vi "STARTUP_.vi"() -> ()   [LabVIEW 2015]
panel:
  out "Current Startup\nAttempt Case - Right 2":i32
  in  "LEFT FOUND":bool
  in  "RIGHT FOUND":bool
  in  "Left Start\nCorrelation Score":dbl
  in  "Right Start\nCorrelation Score":dbl
  out "Current Startup\nAttempt Case - Right":i32
  out "Current Startup\nAttempt Case - Left":i32
  out "Start up Template State\n- LEFT":i32
  in  "Skip Startup - LEFT":bool[](array[boolean])=[FALSE, TRUE, FALSE, FALSE, TRUE, FALSE, FALSE, TRUE]
  in  "Skip Startup - RIGHT":bool[](array[boolean])=[TRUE, TRUE, FALSE, FALSE, FALSE, FALSE, FALSE, FALSE]
  in  "Startup GP per Case - LEFT":u16[](array[numeric])=[920, 0, 260, 700, 0, 200, 650, 0, 358]
  in  "Startup GP per Case - RIGHT":u16[](array[numeric])=[0, 0, 360, 830, 130, 340, 790, 0]
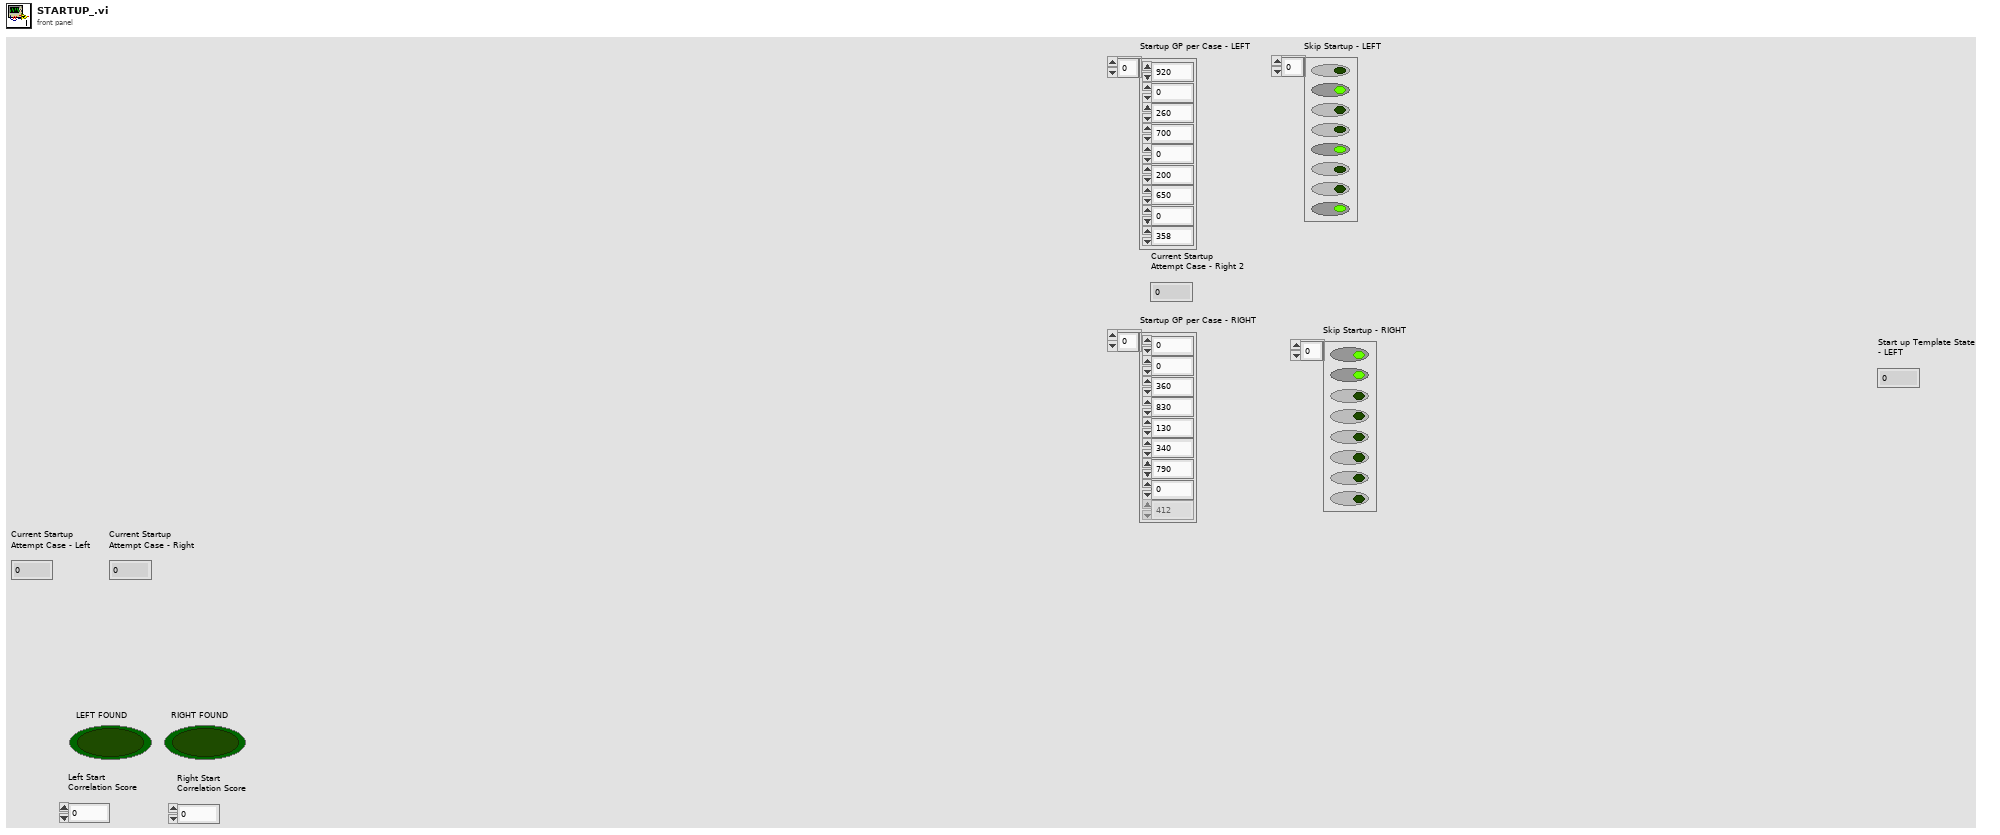
[diagram p1: front panel]
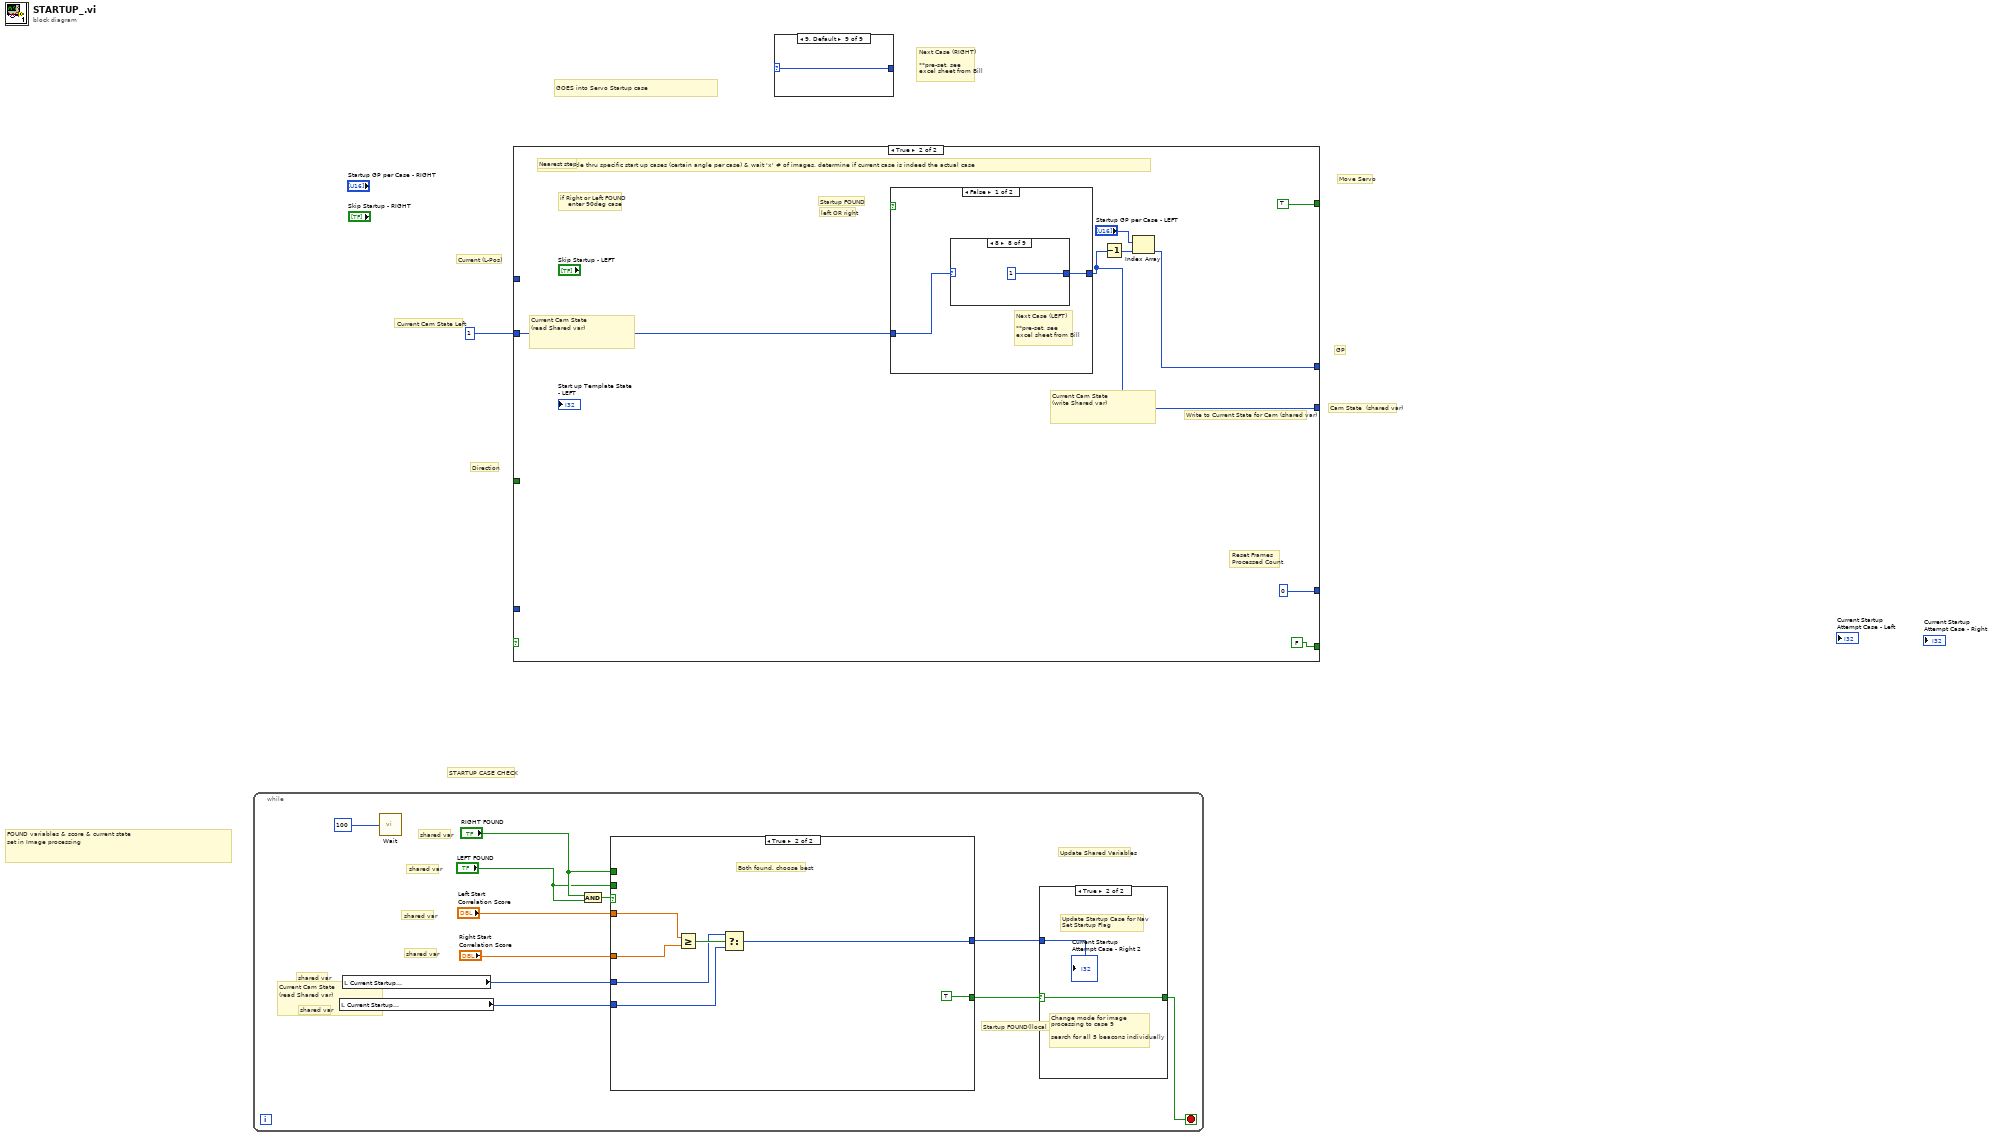
[diagram p0: block diagram]
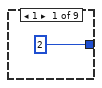
[diagram p2: hidden frame]
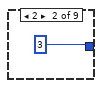
[diagram p3: hidden frame]
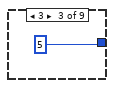
[diagram p4: hidden frame]
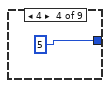
[diagram p5: hidden frame]
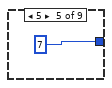
[diagram p6: hidden frame]
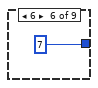
[diagram p7: hidden frame]
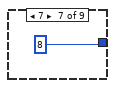
[diagram p8: hidden frame]
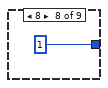
[diagram p9: hidden frame]
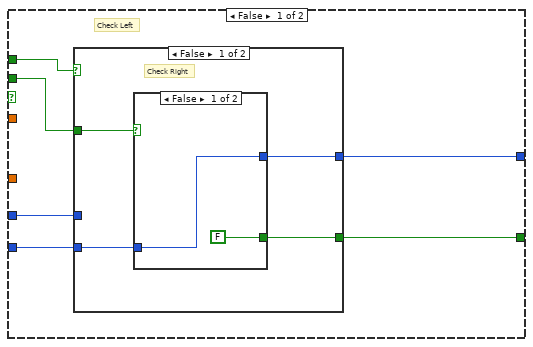
[diagram p11: hidden frame]
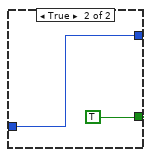
[diagram p12: hidden frame]
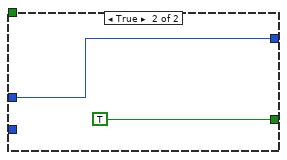
[diagram p13: hidden frame]
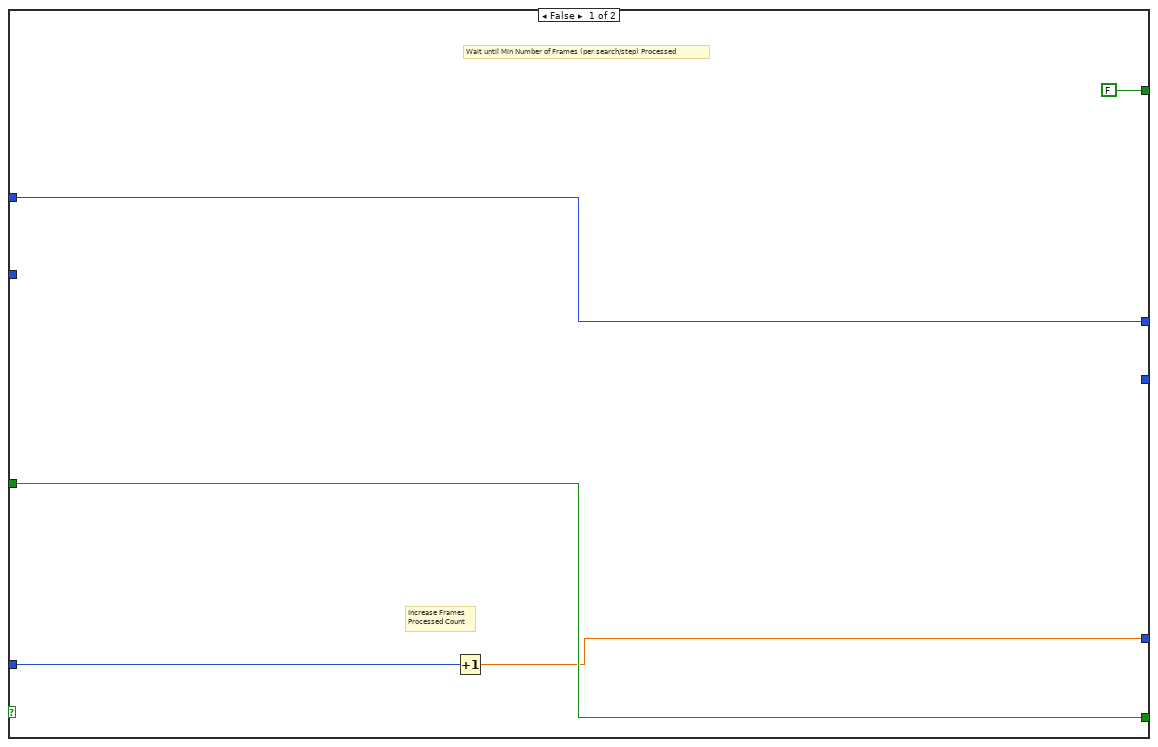
[diagram p14: hidden frame]
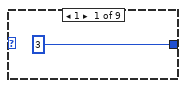
[diagram p15: hidden frame]
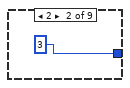
[diagram p16: hidden frame]
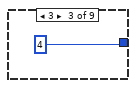
[diagram p17: hidden frame]
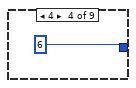
[diagram p18: hidden frame]
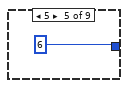
[diagram p19: hidden frame]
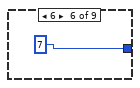
[diagram p20: hidden frame]
diagram:
  # "Next Case (RIGHT)\n\n**pre-set, see\nexcel sheet from Bill"
  # "Cam State  (shared var)"
  # "FOUND variables & score & current state\nset in Image processing"
  # "GOES into Servo Startup case"
  # "STARTUP CASE CHECK"
  # "GP"
  # "Move Servo"
  # "Current Cam State Left"
  # "Direction"
  # "Current (L-Pos)"
  n1 = while {
    stop <- w2 stop-if-true
    # "Startup FOUND(llocal var)"
    # "Current Cam State\n(read Shared var)"
    # "shared var"
    # "shared var"
    # "shared var"
    # "shared var"
    # "shared var"
    # "shared var"
    # "Update Shared Variables"
    n2 = local read "Current Startup\nAttempt Case - Right"() -> (w9:i32)
    n3 = local read "Current Startup\nAttempt Case - Left"() -> (w10:i32)
    n4 = call "Wait"("Count(mSec)"=u32 100) -> ()  [unwired: 1 out]
    n5 = And(x="RIGHT FOUND", y="LEFT FOUND") -> (x .and. y?=w8:bool)
    n6 = case shown="True" w8 {
      tunnel: "Left Start\nCorrelation Score" -> [_ w36]
      tunnel: "Right Start\nCorrelation Score" -> [_ w38]
      tunnel: w10 -> [w19 w35]
      tunnel: w9 -> [w17 w34]
      tunnel: [w20 w33] -> w4
      tunnel: "RIGHT FOUND" -> [w21 _]
      tunnel: "LEFT FOUND" -> [w18 _]
      tunnel: [w16 TRUE] -> w5
      frame False {
        # "Check Left"
        n7 = case shown="False" w21 {
          tunnel: [w24 w31] -> w20
          tunnel: w19 -> [_ w31]
          tunnel: w18 -> [w25 _]
          tunnel: w17 -> [w23 _]
          tunnel: [w22 TRUE] -> w16
          frame False {
            # "Check Right"
            n8 = case shown="False" w25 {
              tunnel: [w26 w29] -> w24
              tunnel: w23 -> [w26 w29]
              tunnel: [FALSE TRUE] -> w22
              frame False {
              }
              frame True {
              }
            }
          }
          frame True {
          }
        }
      }
      frame True {
        # "Both found, choose best"
        n9 = Greater Or Equal?(x=w36, y=w38) -> (x >= y?=w37:bool)
        n10 = Select(t=w35, s=w37, f=w34) -> (s? t:f=w33:i32)
      }
    }
    n11 = case shown="True" w5 {
      selector: w5 -> [w13 w15]
      tunnel: w4 -> [_ w14]
      tunnel: [w13 w15] -> w2
      frame False {
        # "Do nothing"
      }
      frame True {
        # "Change mode for image\nprocessing to case 9\n\nsearch for all 5 beacons individually"
        # "Update Startup Case for Nav\nSet Startup Flag"
        "Current Startup\nAttempt Case - Right 2" <- w14
      }
    }
  }
  n12 = case shown="True" {
    selector: _ -> [_ _]
    tunnel: _ -> [w41 _]
    tunnel: _ -> [w40 _]
    tunnel: [w41 w45] -> _
    tunnel: [w39 0] -> _
    tunnel: [FALSE TRUE] -> _
    tunnel: _ -> [w42 _]
    tunnel: [w40 FALSE] -> _
    tunnel: 1 -> [_ w48]
    tunnel: [_ w44] -> _
    frame False {
      # "Wait until Min Number of Frames (per search/step) Processed"
      # "Increase Frames\nProcessed Count"
      n13 = Increment(x=w42) -> (x+1=w39:dbl)
    }
    frame True {
      # "left OR right"
      # "Startup FOUND"
      # "Current Cam State\n(write Shared var)"
      # "Current Cam State\n(read Shared var)"
      # "Write to Current State for Cam (shared var)"
      # "if Right or Left FOUND\n    enter 90deg case"
      # "Reset Frames\nProcessed Count"
      # "Startup - Cycle thru specific start up cases (certain angle per case) & wait 'x' # of images, determine if current case is indeed the actual case"
      # "Nearest step"
      n14 = case shown="False" {
        selector: _ -> [_ _]
        tunnel: w48 -> [w53 _]
        tunnel: [w52 9] -> w44
        frame False {
          # "Next Case (LEFT)\n\n**pre-set, see\nexcel sheet from Bill"
          n15 = case shown="8" w53 {
            selector: w53 -> [_ _ _ _ _ _ _ _ w62]
            tunnel: [3 3 4 6 6 7 1 1 w62] -> w52
            frame 1 {
            }
            frame 2 {
            }
            frame 3 {
            }
            frame 4 {
            }
            frame 5 {
            }
            frame 6 {
            }
            frame 7 {
            }
            frame 8 {
            }
            frame 9, Default {
              # "stay in 9"
            }
          }
        }
        frame True {
          # "Change mode for image\nprocessing to case 9\n\nsearch for all 5 beacons individually"
          # "Update Startup Case for Nav\nSet Startup Flag"
        }
      }
      n16 = Decrement(x=w44) -> (x-1=w47:i32)
      n17 = Index Array(array="Startup GP per Case - LEFT", index=w47) -> (element=w45:u16)
    }
  }
  n18 = case shown="9, Default" {
    selector: _ -> [_ _ _ _ _ _ _ _ w72]
    tunnel: [2 3 5 5 7 7 8 1 w72] -> _
    frame 1 {
    }
    frame 2 {
    }
    frame 3 {
    }
    frame 4 {
    }
    frame 5 {
    }
    frame 6 {
    }
    frame 7 {
    }
    frame 8 {
    }
    frame 9, Default {
    }
  }
